vi "MosbusRequestSubVI.vi"(1 "Quantity":u8, 2 "Function Code":u8, 3 "Address":u8) -> (0 "String":string)   [LabVIEW 2016]
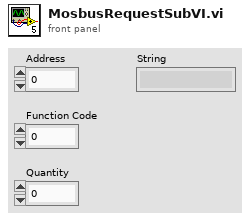
[diagram p1: front panel]
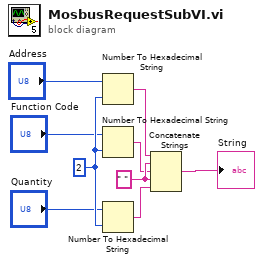
[diagram p0: block diagram]
diagram:
  w8 = i16 2 ("width (-)")
  w6 = " "
  n1 = Number To Hexadecimal String(1:w8, 2:"Address") -> (0:w4:string)
  n2 = Number To Hexadecimal String(1:w8, 2:"Function Code") -> (0:w5:string)
  n3 = Number To Hexadecimal String(1:w8, 2:"Quantity") -> (0:w7:string)
  n4 = Concatenate Strings(w4, w6, w5, w6, w7) -> (→"String":string)
